vi "PH_SHS_Analysis.constructor.vi"(0 "name":string, 2 "data in":string, 5 "error in(no error)":errorcluster) -> (14 "i ref out":refnum<vi>, 16 "data out":string, 19 "error out":errorcluster)   [LabVIEW 2014, in "PH_SHS_Analysis.lvlib"]
doc: "This is the constructor of a class.\n\nLicense Agreement for this software:\n\nCopyright (C)\nGesellschaft für Schwerionenforschung, GSI\nPlanckstr. 1\n64291 Darmstadt\nGermany\n\nContact: D.Beck@gsi.de \n\nThis program is free software; you can redistribute it and/or modify it under the terms of the \nGNU General Public License as published by the Free Software Foundation; either version 2 of \nthe license, or (at your option) any later version.\n\nThis program is distributed in the hope that it will be useful, but WITHOUT ANY WARRANTY; \nwithout even the implied warranty of MERCHANTABILITY or FITNESS FOR A PARTICULAR PURPOSE. See the GNU General License for more details (http://www.gnu.org).\n\nGesellschaft für Schwerionenforschung, GSI\nPlanckstr. 1, 64291 Darmstadt, Germany\nFor all questions and ideas contact: M.Richter@gsi.de, H.Brand@gsi.de or D.Beck@gsi.de.\nLast update: 16-JUN-2004"
uses:
  PH_SHS_Analysis.lvlib
  User/Eisenbarth/SHS_v4/SHS_Analysis/SHS_DeviceConfig.ctl
  PH_Img_BaseClass/PH_Img_BaseClass.Palette.ctl
  CSCore/CSSystem/CSSystemLib/CSSystemLib.lvlib
  PH_PSDBWriter/PH_PSDBWriter.lvlib
  CSCore/BaseProcess/BaseProcess.lvlib
  User/Eisenbarth/SHS_v4/SHS_Analysis/SHS_Analysis.lvlib
  PH_Img_BaseClass/PH_Img_BaseClass.lvlib
  PH_Class/PH_Class.lvlib
  PH_Common/PH_Common.lvlib
  PH_SHS_Analysis_Calibrator/PH_SHS_Analysis_Calibrator.lvlib
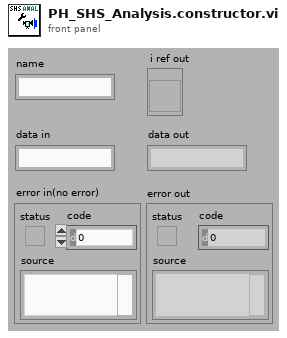
[diagram p1: front panel]
types:
  T1 = enum16{"SetAttribute", "GetAttribute", "CreateAttribute", "DestroyAttribute", "DestroyAllAtributes"}
  T2 = typedef "SHS_Analysis.lvlib/SHS_DeviceConfig.ctl" = cluster{"focal length [m]":dbl, "pixel size [m/px]":dbl, "wavelength [m]":dbl}
  T3 = typedef "PH_Img_BaseClass.lvlib/PH_Img_BaseClass.Palette.ctl" = i32
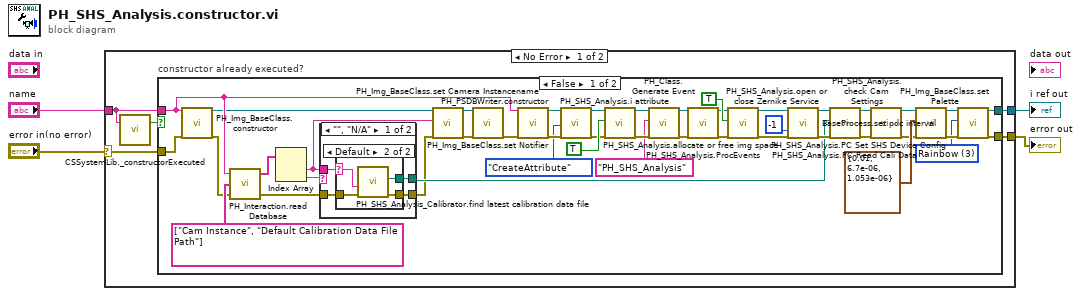
[diagram p0: block diagram]
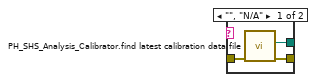
[diagram p2: hidden frame]
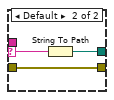
[diagram p3: hidden frame]
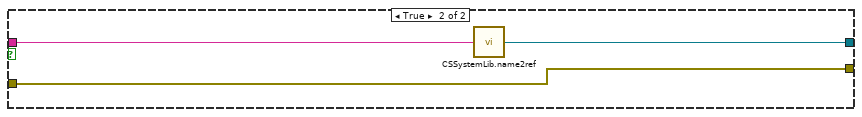
[diagram p4: hidden frame]
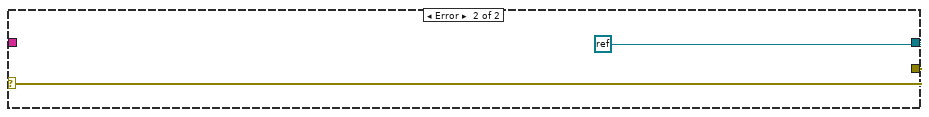
[diagram p5: hidden frame]
diagram:
  n1 = case shown="No Error" "error in(no error)" {
    selector: "error in(no error)" -> [w7 w70]
    tunnel: "name" -> [w6 _]
    tunnel: [w9 refnum<k0> refnum] -> w3
    tunnel: [w8 w70] -> w2
    frame No Error {
      n2 = call "CSSystemLib._constructorExecuted.vi"("name"=w6) -> ("constructor executed?"=w5:bool)  [unwired: 18 in]
      n3 = case "constructor already executed?" shown="False" w5 {
        tunnel: [w22 w68] -> w9
        tunnel: [w21 w67] -> w8
        tunnel: w7 -> [w52 w67]
        tunnel: w6 -> [w18 w69]
        frame False {
          w40 = T3 3 items=["Grey", "Binary", "Gradient", "Rainbow", "Temperature"] ("Palette")
          n4 = call "PH_Img_BaseClass.constructor.vi"("name"=w18, "error in(no error)"=w52) -> ("i ref out"=w12:refnum<vi>, "error out"=w11:errorcluster)  [unwired: 15 in, 1 out]
          n5 = call "PH_Interaction.read Database.vi"("error in (no error)"=w11, "Strings to search for"=string[] ["Cam Instance", "Default Calibration Data File Path"], "DB Entry to read"=w18) -> ("error out"=w16:errorcluster, "Values"=w17:string[])  [unwired: 1 in]
          n6 = Index Array(array=w17) -> (element #1=w14:string, element #2=w15:string)  [unwired: 2 in]
          n7 = case shown="\"\", \"N/A\"" w15 {
            selector: w15 -> [_ w65]
            tunnel: [w56 w66] -> w13
            tunnel: w14 -> [w53 _]
            tunnel: w16 -> [w55 w64]
            tunnel: [w54 w64] -> w10
            frame "", "N/A" {
              n8 = case shown="Default" w53 {
                selector: w53 -> [_ w60]
                tunnel: [w57 w63] -> w56
                tunnel: w55 -> [w59 w62]
                tunnel: [w58 w61] -> w54
                frame "", "N/A" {
                  n9 = call "PH_SHS_Analysis_Calibrator.find latest calibration data file.vi"("error in (no error)"=w59) -> ("error out"=w58:errorcluster, "latest file"=w57:path)  [unwired: 4 in, 1 out]
                }
                frame Default {
                  n10 = call "PH_SHS_Analysis_Calibrator.find latest calibration data file.vi"("error in (no error)"=w62, "Certain Camera Instance?"=w60) -> ("error out"=w61:errorcluster, "latest file"=w63:path)  [unwired: 3 in, 1 out]
                }
              }
            }
            frame Default {
              n11 = String To Path(string=w65) -> (path=w66:path)
            }
          }
          n12 = call "PH_Img_BaseClass.set Camera Instancename.vi"("i ref in"=w12, "Camera Instancename"=w14, "error in (no error)"=w10) -> ("i ref out"=w43:refnum<vi>, "error out"=w42:errorcluster)  [unwired: 15 in]
          n13 = call "PH_Img_BaseClass.set Notifier.vi"("i ref in"=w43, "error in"=w42) -> ("error out"=w20:errorcluster)  [unwired: 16 in, 1 out]
          n14 = call "PH_PSDBWriter.constructor.vi"("name"=w18, "error in"=w20) -> ("i ref out"=w34:refnum<vi>, "error out"=w33:errorcluster)  [unwired: 15 in, 1 out]
          n15 = call "PH_SHS_Analysis.i attribute.vi"("VI Refnum"=w34, "Action"=T1."CreateAttribute", "error in (no error)"=w33) -> ("VI Refnum out"=w35:refnum<vi>, "error out"=w36:errorcluster)  [unwired: 14 in, 1 out]
          n16 = call "PH_SHS_Analysis.allocate or free img space.vi"("i ref in"=w35, "Allocate?"=TRUE, "error in (no error)"=w36) -> ("i ref out"=w31:refnum<vi>, "error out"=w32:errorcluster)  [unwired: 15 in]
          n17 = call "PH_Class.Generate Event.vi"("i ref in"=w31, "Class"="PH_SHS_Analysis", "error in (no error)"=w32) -> ("i ref out"=w39:refnum<vi>, "error out"=w38:errorcluster)  [unwired: 15 in]
          n18 = call "PH_SHS_Analysis.ProcEvents.vi"("i ref in"=w39, "error in"=w38) -> ("i ref out"=w28:refnum<vi>, "error out"=w27:errorcluster)  [unwired: 16 in]
          n19 = call "PH_SHS_Analysis.open or close Zernike Service.vi"("i ref in"=w28, "open"=TRUE, "error in (no error)"=w27) -> ("i ref out"=w26:refnum<vi>, "error out"=w25:errorcluster)  [unwired: 15 in]
          n20 = call "BaseProcess.set pdc interval.vi"("i ref in"=w26, "PeriodicInterval [ms]"=-1 ("PeriodicInterval"), "error in (no error)"=w25) -> ("i ref out"=w24:refnum<vi>, "error out"=w23:errorcluster)  [unwired: 14 in, 1 out]
          n21 = call "PH_SHS_Analysis.PC Read Cali Data.vi"("i ref in"=w24, "Cali Data File"=w13, "error in (no error)"=w23) -> ("i ref out"=w50:refnum<vi>, "error out"=w49:errorcluster)  [unwired: 15 in]
          n22 = call "PH_SHS_Analysis.check Cam Settings.vi"("i ref in"=w50, "error in"=w49) -> ("i ref out"=w45:refnum<vi>, "error out"=w44:errorcluster)  [unwired: 16 in]
          n23 = call "PH_SHS_Analysis.PC Set SHS Device Config.vi"("i ref in"=w45, "SHS Device Config"=T2 {"focal length [m]"=0.01, "pixel size [m/px]"=6.7e-06, "wavelength [m]"=1.053e-06}, "error IO"=w44) -> ("i ref out"=w41:refnum<vi>, "error out"=w47:errorcluster)  [unwired: 15 in]
          n24 = call "PH_Img_BaseClass.set Palette.vi"("i ref in"=w41, "Palette"=w40, "error in (no error)"=w47) -> ("i ref out"=w22:refnum<vi>, "error out"=w21:errorcluster)  [unwired: 15 in]
        }
        frame True {
          n25 = call "CSSystemLib.name2ref.vi"("name"=w69) -> ("obj refnum"=w68:refnum<vi>)
        }
      }
    }
    frame Error {
    }
  }
  "i ref out" <- w3
  "error out" <- w2
